vi "Watcher Loop Async.vi"(11 "App Watcher in":refnum<class "App Watcher.lvclass">) -> ()   [LabVIEW 2020, in "PicoG-App.lvlib" / "App Watcher.lvclass"]
uses:
  App Watcher.lvclass
  App Watcher.lvclass/App Watcher.ctl
panel:
  # "App Watcher"
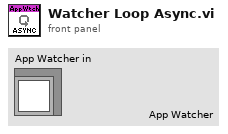
[diagram p1: front panel]
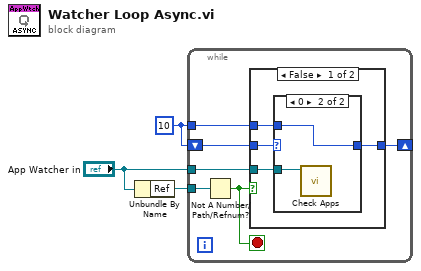
[diagram p0: block diagram]
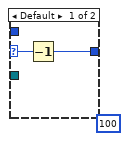
[diagram p2: hidden frame]
diagram:
  w1 = 10
  n1 = Unbundle By Name("App Watcher in") -> ("Ref"=w3:refnum<data-value>)
  n2 = while {
    tunnel: w3 -> [w7]
    shift-right: [w5] -> _
    shift-left: w1 -> [w9]
    tunnel: "App Watcher in" -> [w6]
    tunnel: w1 -> [w4]
    stop <- w8 stop-if-true
    n3 = Not A Number/Path/Refnum?(number/path/refnum=w7) -> (NaN/Path/Refnum?=w8:bool)
    n4 = case shown="False" w8 {
      tunnel: w9 -> [w12 w19]
      tunnel: w6 -> [w13 _]
      tunnel: [w11 w19] -> w5
      tunnel: w4 -> [w10 _]
      frame False {
        n5 = case shown="0" w12 {
          selector: w12 -> [w16 _]
          tunnel: w13 -> [_ w18]
          tunnel: [w15 w17] -> w11
          tunnel: w10 -> [_ w17]
          frame Default {
            n6 = Decrement(x=w16) -> (x-1=w15:i32)
            n7 = Wait (ms)(milliseconds to wait=u32 100) -> ()  [unwired: 1 out]
          }
          frame 0 {
            n8 = call "Check Apps.vi"("App Watcher in"=w18) -> ()  [unwired: 11 in]
          }
        }
      }
      frame True {
      }
    }
  }
